vi "Signal.Convert.StringArray.vi"(8 "error in (no error)":errorcluster, 11 "Signal Parameters":string[](array[string])) -> (0 "error out":errorcluster, 3 "Signal Parameters":T1 {"Byte Order" items=["Little Endian", "Big Endian"]; "Data Type" items=["Signed", "Unsigned", "IEEE Float"]})   [LabVIEW 2019, in "Diagnostics Addon System Explorer.lvlib"]
uses:
  Diagnostics Addon System Explorer.lvlib
  Addon Shared/Types/Signal.ctl
  Addon Shared/Diagnostics Addon Shared.lvlib
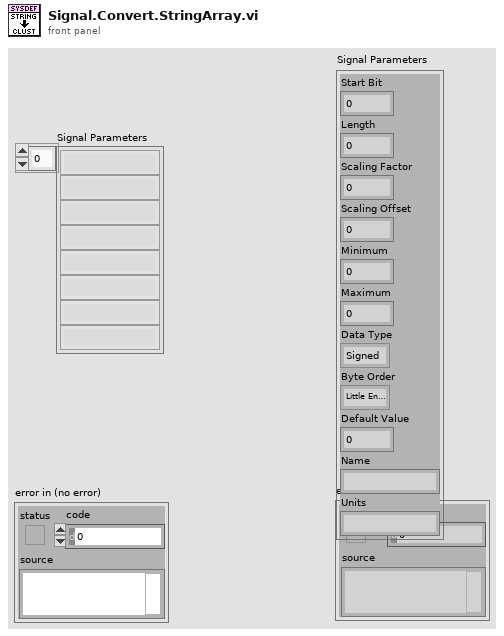
[diagram p1: front panel]
types:
  T1 = typedef "Diagnostics Addon Shared.lvlib/Signal.ctl" = cluster{"Start Bit":u32, "Length":u32, "Scaling Factor":dbl, "Scaling Offset":dbl, "Minimum":dbl, "Maximum":dbl, "Data Type":u32, "Byte Order":u32, "Default Value":dbl, "Name":string, "Units":string}
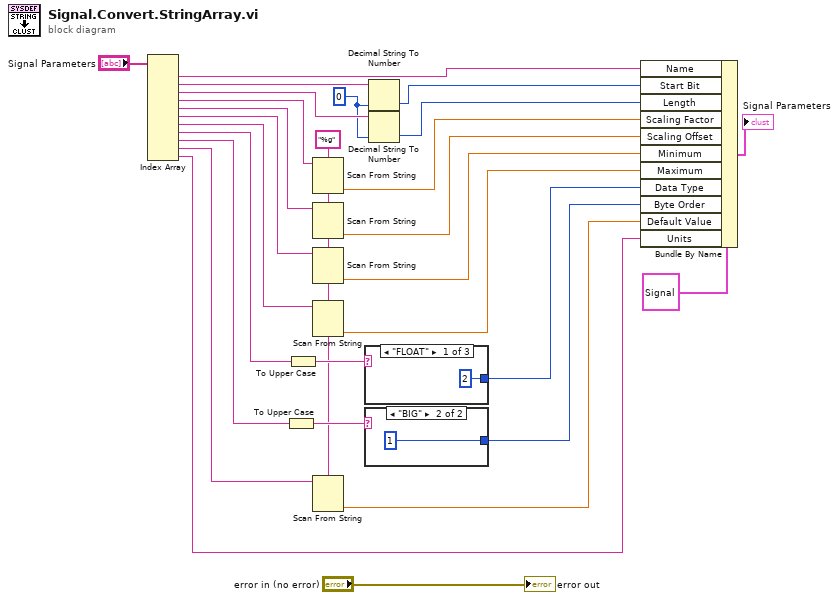
[diagram p0: block diagram]
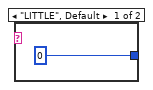
[diagram p2: hidden frame]
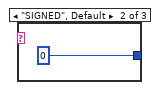
[diagram p3: hidden frame]
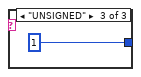
[diagram p4: hidden frame]
diagram:
  w1 = "%g" ("format string")
  w22 = u32 0 ("Start Bit")
  n1 = Index Array(array="Signal Parameters") -> (element #1=w25:string, element #2=w24:string, element #3=w23:string, element #4=w19:string, element #5=w5:string, element #6=w7:string, element #7=w9:string, element #8=w17:string, element #9=w14:string, element #10=w3:string, element #11=w11:string)  [unwired: 11 in]
  n2 = To Upper Case(1:w14) -> (0:w13:string)
  n3 = To Upper Case(1:w17) -> (0:w16:string)
  n4 = Scan From String(format string=w1, input string=w19) -> (output 1=w10:dbl)  [unwired: 3 in, 3 out]
  n5 = Scan From String(format string=w1, input string=w5) -> (output 1=w4:dbl)  [unwired: 3 in, 3 out]
  n6 = Scan From String(format string=w1, input string=w7) -> (output 1=w6:dbl)  [unwired: 3 in, 3 out]
  n7 = Scan From String(format string=w1, input string=w9) -> (output 1=w8:dbl)  [unwired: 3 in, 3 out]
  n8 = Scan From String(format string=w1, input string=w3) -> (output 1=w2:dbl)  [unwired: 3 in, 3 out]
  n9 = case shown="\"FLOAT\"" w16 {
    tunnel: [2 0 1] -> w15
    frame "FLOAT" {
    }
    frame "SIGNED", Default {
    }
    frame "UNSIGNED" {
    }
  }
  n10 = case shown="\"BIG\"" w13 {
    tunnel: [0 1] -> w12
    frame "LITTLE", Default {
    }
    frame "BIG" {
    }
  }
  n11 = Decimal String To Number(string=w24, default (0L)=w22) -> (number=w21:u32)  [unwired: 1 in, 1 out]
  n12 = Decimal String To Number(string=w23, default (0L)=w22) -> (number=w20:u32)  [unwired: 1 in, 1 out]
  n13 = Bundle By Name(cluster=T1 {"Start Bit"=0, "Length"=0, "Scaling Factor"=0.0, "Scaling Offset"=0.0, "Minimum"=0.0, "Maximum"=0.0, "Data Type"=0, "Byte Order"=0, "Default Value"=0.0, "Name"="", "Units"=""} ("Signal Parameters"), "Name"=w25, "Start Bit"=w21, "Length"=w20, "Scaling Factor"=w10, "Scaling Offset"=w4, "Minimum"=w6, "Maximum"=w8, "Data Type"=w15, "Byte Order"=w12, "Default Value"=w2, "Units"=w11) -> (→"Signal Parameters":T1)
  "error out" <- "error in (no error)"
